vi "Camera.vi"() -> ()   [LabVIEW 2016, in "Test2.lvrbt"]
uses:
  Test2.lvrbt
  <vilib>/NXT/LegoClasses/BrickReference/BrickReference.lvclass
  <vilib>/NXT/Subs/LVHSConnector.ctl
  <vilib>/NXT/NXTIO Xnodes/NXTIOXNode/NXTIO.xnode
  <vilib>/NXT/NXTIO Xnodes/AddressXNode/NXTIOAddress.xnode
  <vilib>/NXT/Hardware/Plugins/Tetrix DC Motor/TetrixDCMotorAddress.ctl
  <vilib>/NXT/NXTIO Xnodes/NXTIONodeSubVIs/TETRIX IO Move DC Motors.vi
  <vilib>/NXT/Dual Mode Library/Waits/Wait_EV3_Color_Color.vi
  <vilib>/NXT/Subs/ColorSensorColors.ctl
  <vilib>/NXT/Block Support/NXT_InputPort.ctl
  <vilib>/NXT/NXTIO Xnodes/NXTIONodeSubVIs/TETRIX IO Stop DC Motors.vi
  <vilib>/NXT/Dual Mode Library/Waits/Wait_Num.vi
panel:
  in  "stop":bool
  out "Power":bool
  out "X Upper Left":u8
  out "X Lower Right":u8
  out "Y Lower Right":u8
  out "Y Upper Left":u8
  out "Count":u8
  out "Color":u8
  in  "Cluster":T1 {"Tracking Mode" items=["Disable Tracking", "Get First Object", "Get n th Object", "Enable Tracking", "Sort Objects  by size", "Sort Objects  by Colors", "Illumination on ", "Illumination Off", "Write Colormap", "Read Colormap", "Line tracking mode", "Object Tracking mode"]}
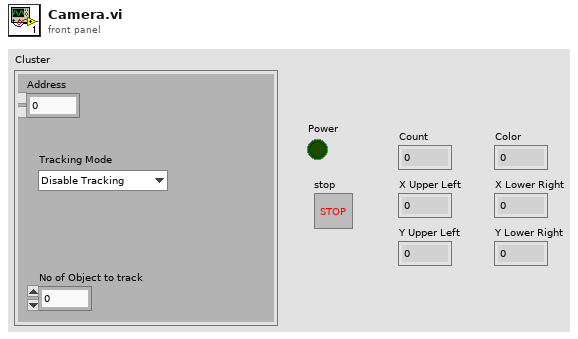
[diagram p1: front panel]
types:
  T1 = cluster{"Address":dbl, "No of Object to track":dbl, "Tracking Mode":u8}
  T2 = cluster{"Tracking Mode":u8, "Object Number to Track":u8, "Address":u8}
  T3 = typedef "NXT_InputPort.ctl" = u32
  T4 = typedef "ColorSensorColors.ctl" = enum16{"No Color", "Black", "Blue", "Green", "Yellow", "Red", "White", "Brown"}
  T5 = typedef "TetrixDCMotorAddress.ctl" = i32
  T6 = typedef "LVHSConnector.ctl" = refnum<class "BrickReference.lvclass">
  T7 = cluster{"TetrixDCMotor":T5, "TetrixDCMotor 2":T5}
  T8 = cluster{"Total Tracked Objects":u8, "Color":u8, "X Upper Left":u8, "Y Upper Left":u8, "X Lower Right":u8, "Y Lower Right":u8, "Status (boolean)":bool}
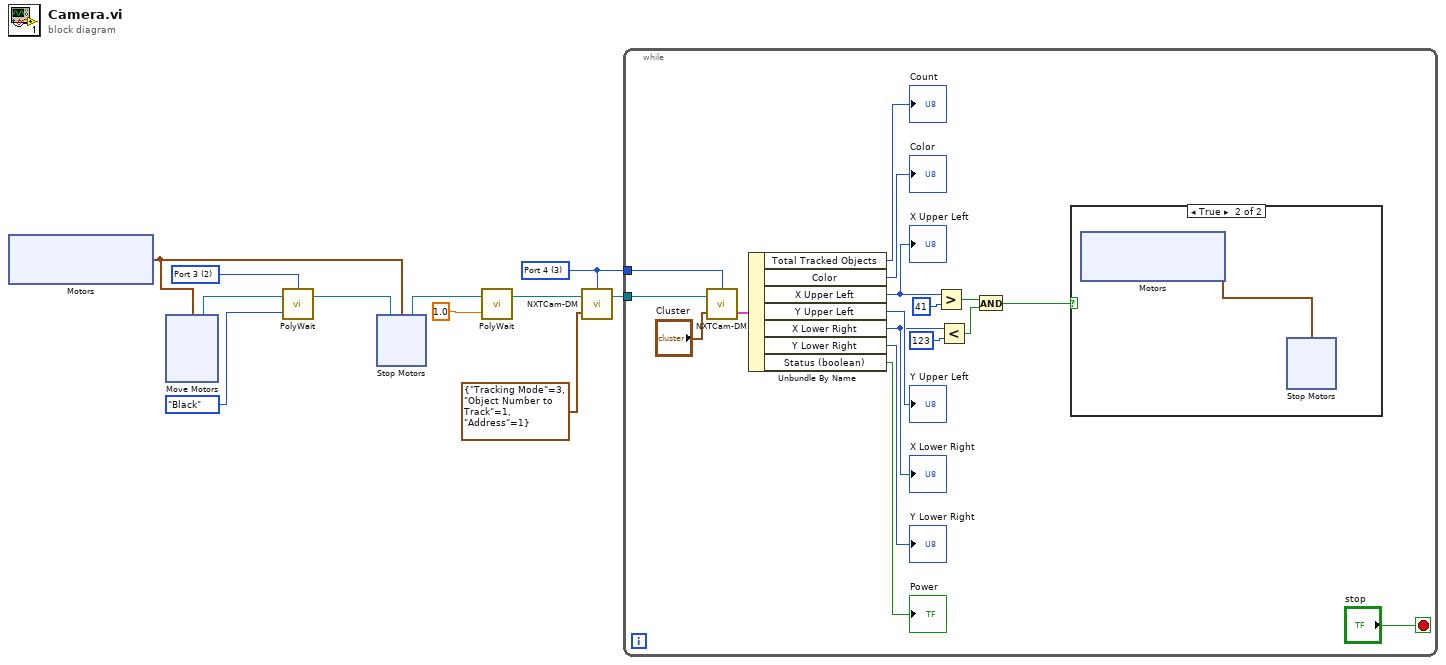
[diagram p0: block diagram]
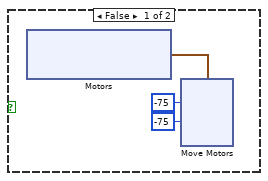
[diagram p2: hidden frame]
diagram:
  w2 = T3 3 items=["Port 1", "Port 2", "Port 3", "Port 4"] ("Input Port")
  w9 = T3 2 items=["Port 1", "Port 2", "Port 3", "Port 4"] ("Port (Port 1)")
  n1 = xnode "Motors"() -> ("Motor"=w7:cluster{"TetrixDCMotor":T5, "TetrixDCMotor":T5})
  n2 = xnode "Move Motors"("Motors"=w7) -> ("NXT/EV3"=w11:T6)  [unwired: 3 in]
  n3 = call-poly <vilib>:"PolyWait.vi"("Color (Red)"=ColorSensorColors."Black", "NXT/EV3"=w11, "Port (Port 1)"=w9) -> ("NXT/EV3"=w8:T6)  [unwired: 1 in]
  n4 = xnode "Stop Motors"("Motors"=w7, "NXT/EV3"=w8) -> ("NXT/EV3"=w6:T6)
  n5 = call-poly <vilib>:"PolyWait.vi"("Time (1 sec)"=sgl 1.0, "NXT/EV3"=w6) -> ("NXT/EV3"=w1:T6)  [unwired: 2 in]
  n6 = call "NXTCam-DM.vi"("Input of NXTCam"=T2 {"Tracking Mode"=3, "Object Number to Track"=1, "Address"=1}, "NXT"=w1, "Input Port"=w2) -> ("NXT dup"=w4:T6)  [unwired: 1 out]
  n7 = while {
    tunnel: w2 -> [w26]
    tunnel: w4 -> [w25]
    stop <- "stop" stop-if-true
    n8 = call "NXTCam-DM.vi"("Input of NXTCam"="Cluster", "NXT"=w25, "Input Port"=w26) -> ("Output of NXTCam"=w21:T8)  [unwired: 1 out]
    n9 = Unbundle By Name(w21) -> ("Total Tracked Objects"=→"Count":u8, "Color"=→"Color":u8, "X Upper Left"=w19:u8, "Y Upper Left"=→"Y Upper Left":u8, "X Lower Right"=w17:u8, "Y Lower Right"=→"Y Lower Right":u8, "Status (boolean)"=→"Power":bool)
    "X Upper Left" <- w19
    "X Lower Right" <- w17
    n10 = Greater?(x=w19, y=u8 41) -> (0:w15:bool)
    n11 = Less?(x=w17, y=u8 123) -> (x < y?=w14:bool)
    n12 = And(x=w15, y=w14) -> (x .and. y?=w13:bool)
    n13 = case shown="True" w13 {
      frame False {
        n14 = xnode "Motors"() -> ("Motor"=w31:cluster{"TetrixDCMotor":T5, "TetrixDCMotor":T5})
        n15 = xnode "Move Motors"("Power/Speed 2"=i8 -75, "Power/Speed 1"=i8 -75, "Motors"=w31) -> ()  [unwired: 1 in, 1 out]
      }
      frame True {
        n16 = xnode "Motors"() -> ("Motor"=w41:cluster{"TetrixDCMotor":T5, "TetrixDCMotor":T5})
        n17 = xnode "Stop Motors"("Motors"=w41) -> ()  [unwired: 1 in, 1 out]
      }
    }
  }
